vi "Remote Time Check SubVI - Evaluate Results.vi"(6 "Tolerance (ms)":u32, 8 "error in (no error)":errorcluster, 9 "Start Tick Count (ms)":u32, 10 "Completion Tick Count (ms)":u32, 11 "Remote Time String (ms)":string) -> (0 "error out":errorcluster, 1 "Remote OS Up Time (ms)":u32, 2 "Windows OS Up Time (ms)":u32, 3 "Valid Trip Time":bool)   [LabVIEW 2010, in "Core SubVIs.lvlib"]
doc: "Compare Start and Completion Tick time differences agains the Tolerance value. If tick count difference is less than tolerance, it is a valid trip time and the Windows OS time is estimated and the Remote Time String is parsed to create the Remote OS Up Time value."
uses:
  Core SubVIs.lvlib
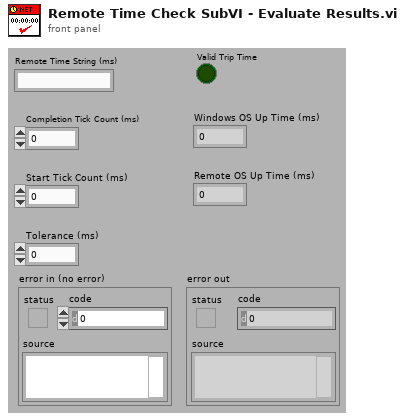
[diagram p1: front panel]
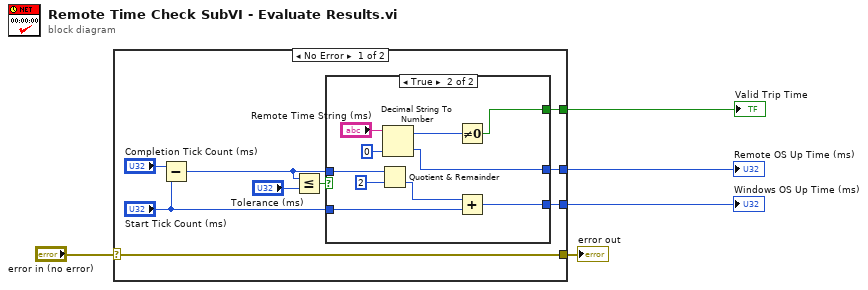
[diagram p0: block diagram]
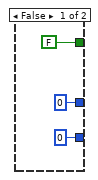
[diagram p2: hidden frame]
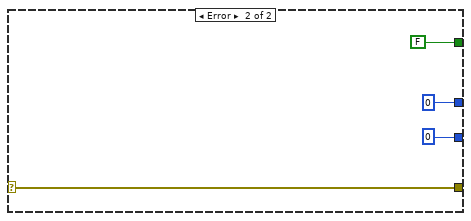
[diagram p3: hidden frame]
diagram:
  n1 = case shown="No Error" "error in (no error)" {
    selector: "error in (no error)" -> [w12 w28]
    tunnel: [w12 w28] -> w4
    tunnel: [w9 u32 0 ("Mac OS Up Time (ms)")] -> w3
    tunnel: [w6 u32 0 ("Windows OS Up Time (ms)")] -> w2
    tunnel: [w10 FALSE] -> w1
    frame No Error {
      n2 = Subtract(x="Completion Tick Count (ms)", y="Start Tick Count (ms)") -> (x-y=w8:u32)
      n3 = Less Or Equal?(x=w8, y="Tolerance (ms)") -> (x <= y?=w11:bool)
      n4 = case shown="True" w11 {
        tunnel: [FALSE w18] -> w10
        tunnel: [u32 0 w25] -> w9
        tunnel: w8 -> [_ w24]
        tunnel: "Start Tick Count (ms)" -> [_ w22]
        tunnel: [u32 0 w20] -> w6
        frame False {
        }
        frame True {
          n5 = Quotient & Remainder(x=w24, y=u32 2) -> (floor(x/y)=w21:u32)  [unwired: 1 out]
          n6 = Decimal String To Number(string="Remote Time String (ms)", default (0L)=u32 0 ("default (0 I32)")) -> (offset past number=w19:i32, number=w25:u32)  [unwired: 1 in]
          n7 = Not Equal To 0?(x=w19) -> (x != 0?=w18:bool)
          n8 = Add(x=w21, y=w22) -> (x+y=w20:u32)
        }
      }
    }
    frame Error {
    }
  }
  "Windows OS Up Time (ms)" <- w2
  "Remote OS Up Time (ms)" <- w3
  "error out" <- w4
  "Valid Trip Time" <- w1
